vi "App - analyze RUS V6.vi"() -> ()   [LabVIEW 2021] (continued)
"last mod"=timestamp(3493899198 s since 1904-01-01), "file name str"="D:\\Data\\Ultrasound\\LSCO\\LSCO22__130814c\\5_Cooling_2nd_try\\September_2014\\091814\\14.78800K_500_2500_2.10000V_0.00000T_Sep18-2014__11-33-18_001_091814.bin", "mod time(min)"=58231653.3, "file format"=enum."binary", "power(V)"=2.1, "Magn Field(T) "=0.0}, {"temperature"=14.791, "temperature str"="14.79100", "file path"=path "D:/Data/Ultrasound/LSCO/LSCO22__130814c/5_Cooling_2nd_try/September_2014/091814/14.79100K_500_2500_2.10000V_0.00000T_Sep18-2014__11-34-37_001_091814.bin", "last mod"=timestamp(3493899277 s since 1904-01-01), "file name str"="D:\\Data\\Ultrasound\\LSCO\\LSCO22__130814c\\5_Cooling_2nd_try\\September_2014\\091814\\14.79100K_500_2500_2.10000V_0.00000T_Sep18-2014__11-34-37_001_091814.bin", "mod time(min)"=58231654.61666667, "file format"=enum."binary", "power(V)"=2.1, "Magn Field(T) "=0.0}, {"temperature"=14.793, "temperature str"="14.79300", "file path"=path "D:/Data/Ultrasound/LSCO/LSCO22__130814c/5_Cooling_2nd_try/September_2014/091814/14.79300K_500_2500_2.10000V_0.00000T_Sep18-2014__11-35-56_001_091814.bin", "last mod"=timestamp(3493899356 s since 1904-01-01), "file name str"="D:\\Data\\Ultrasound\\LSCO\\LSCO22__130814c\\5_Cooling_2nd_try\\September_2014\\091814\\14.79300K_500_2500_2.10000V_0.00000T_Sep18-2014__11-35-56_001_091814.bin", "mod time(min)"=58231655.93333333, "file format"=enum."binary", "power(V)"=2.1, "Magn Field(T) "=0.0}, {"temperature"=14.796, "temperature str"="14.79600", "file path"=path "D:/Data/Ultrasound/LSCO/LSCO22__130814c/5_Cooling_2nd_try/September_2014/091814/14.79600K_500_2500_2.10000V_0.00000T_Sep18-2014__11-37-16_001_091814.bin", "last mod"=timestamp(3493899436 s since 1904-01-01), "file name str"="D:\\Data\\Ultrasound\\LSCO\\LSCO22__130814c\\5_Cooling_2nd_try\\September_2014\\091814\\14.79600K_500_2500_2.10000V_0.00000T_Sep18-2014__11-37-16_001_091814.bin", "mod time(min)"=58231657.266666666, "file format"=enum."binary", "power(V)"=2.1, "Magn Field(T) "=0.0}, {"temperature"=14.797, "temperature str"="14.79700", "file path"=path "D:/Data/Ultrasound/LSCO/LSCO22__130814c/5_Cooling_2nd_try/September_2014/091814/14.79700K_500_2500_2.10000V_0.00000T_Sep18-2014__11-38-35_001_091814.bin", "last mod"=timestamp(3493899515 s since 1904-01-01), "file name str"="D:\\Data\\Ultrasound\\LSCO\\LSCO22__130814c\\5_Cooling_2nd_try\\September_2014\\091814\\14.79700K_500_2500_2.10000V_0.00000T_Sep18-2014__11-38-35_001_091814.bin", "mod time(min)"=58231658.583333336, "file format"=enum."binary", "power(V)"=2.1, "Magn Field(T) "=0.0}, {"temperature"=14.8, "temperature str"="14.80000", "file path"=path "D:/Data/Ultrasound/LSCO/LSCO22__130814c/5_Cooling_2nd_try/September_2014/091814/14.80000K_500_2500_2.10000V_0.00000T_Sep18-2014__11-39-54_001_091814.bin", "last mod"=timestamp(3493899594 s since 1904-01-01), "file name str"="D:\\Data\\Ultrasound\\LSCO\\LSCO22__130814c\\5_Cooling_2nd_try\\September_2014\\091814\\14.80000K_500_2500_2.10000V_0.00000T_Sep18-2014__11-39-54_001_091814.bin", "mod time(min)"=58231659.9, "file format"=enum."binary", "power(V)"=2.1, "Magn Field(T) "=0.0}, {"temperature"=14.807, "temperature str"="14.80700", "file path"=path "D:/Data/Ultrasound/LSCO/LSCO22__130814c/5_Cooling_2nd_try/September_2014/091814/14.80700K_500_2500_2.10000V_0.00000T_Sep18-2014__11-41-14_001_091814.bin", "last mod"=timestamp(3493899674 s since 1904-01-01), "file name str"="D:\\Data\\Ultrasound\\LSCO\\LSCO22__130814c\\5_Cooling_2nd_try\\September_2014\\091814\\14.80700K_500_2500_2.10000V_0.00000T_Sep18-2014__11-41-14_001_091814.bin", "mod time(min)"=58231661.233333334, "file format"=enum."binary", "power(V)"=2.1, "Magn Field(T) "=0.0}, {"temperature"=14.806, "temperature str"="14.80600", "file path"=path "D:/Data/Ultrasound/LSCO/LSCO22__130814c/5_Cooling_2nd_try/September_2014/091814/14.80600K_500_2500_2.10000V_0.00000T_Sep18-2014__11-42-33_001_091814.bin", "last mod"=timestamp(3493899753 s since 1904-01-01), "file name str"="D:\\Data\\Ultrasound\\LSCO\\LSCO22__130814c\\5_Cooling_2nd_try\\September_2014\\091814\\14.80600K_500_2500_2.10000V_0.00000T_Sep18-2014__11-42-33_001_091814.bin", "mod time(min)"=58231662.55, "file format"=enum."binary", "power(V)"=2.1, "Magn Field(T) "=0.0}, {"temperature"=14.808, "temperature str"="14.80800", "file path"=path "D:/Data/Ultrasound/LSCO/LSCO22__130814c/5_Cooling_2nd_try/September_2014/091814/14.80800K_500_2500_2.10000V_0.00000T_Sep18-2014__11-43-53_001_091814.bin", "last mod"=timestamp(3493899833 s since 1904-01-01), "file name str"="D:\\Data\\Ultrasound\\LSCO\\LSCO22__130814c\\5_Cooling_2nd_try\\September_2014\\091814\\14.80800K_500_2500_2.10000V_0.00000T_Sep18-2014__11-43-53_001_091814.bin", "mod time(min)"=58231663.88333333, "file format"=enum."binary", "power(V)"=2.1, "Magn Field(T) "=0.0}, {"temperature"=14.812, "temperature str"="14.81200", "file path"=path "D:/Data/Ultrasound/LSCO/LSCO22__130814c/5_Cooling_2nd_try/September_2014/091814/14.81200K_500_2500_2.10000V_0.00000T_Sep18-2014__11-45-12_001_091814.bin", "last mod"=timestamp(3493899912 s since 1904-01-01), "file name str"="D:\\Data\\Ultrasound\\LSCO\\LSCO22__130814c\\5_Cooling_2nd_try\\September_2014\\091814\\14.81200K_500_2500_2.10000V_0.00000T_Sep18-2014__11-45-12_001_091814.bin", "mod time(min)"=58231665.2, "file format"=enum."binary", "power(V)"=2.1, "Magn Field(T) "=0.0}, {"temperature"=14.814, "temperature str"="14.81400", "file path"=path "D:/Data/Ultrasound/LSCO/LSCO22__130814c/5_Cooling_2nd_try/September_2014/091814/14.81400K_500_2500_2.10000V_0.00000T_Sep18-2014__11-46-31_001_091814.bin", "last mod"=timestamp(3493899991 s since 1904-01-01), "file name str"="D:\\Data\\Ultrasound\\LSCO\\LSCO22__130814c\\5_Cooling_2nd_try\\September_2014\\091814\\14.81400K_500_2500_2.10000V_0.00000T_Sep18-2014__11-46-31_001_091814.bin", "mod time(min)"=58231666.516666666, "file format"=enum."binary", "power(V)"=2.1, "Magn Field(T) "=0.0}, {"temperature"=14.82, "temperature str"="14.82000", "file path"=path "D:/Data/Ultrasound/LSCO/LSCO22__130814c/5_Cooling_2nd_try/September_2014/091814/14.82000K_500_2500_2.10000V_0.00000T_Sep18-2014__11-47-51_001_091814.bin", "last mod"=timestamp(3493900071 s since 1904-01-01), "file name str"="D:\\Data\\Ultrasound\\LSCO\\LSCO22__130814c\\5_Cooling_2nd_try\\September_2014\\091814\\14.82000K_500_2500_2.10000V_0.00000T_Sep18-2014__11-47-51_001_091814.bin", "mod time(min)"=58231667.85, "file format"=enum."binary", "power(V)"=2.1, "Magn Field(T) "=0.0}, {"temperature"=14.816, "temperature str"="14.81600", "file path"=path "D:/Data/Ultrasound/LSCO/LSCO22__130814c/5_Cooling_2nd_try/September_2014/091814/14.81600K_500_2500_2.10000V_0.00000T_Sep18-2014__11-49-10_001_091814.bin", "last mod"=timestamp(3493900150 s since 1904-01-01), "file name str"="D:\\Data\\Ultrasound\\LSCO\\LSCO22__130814c\\5_Cooling_2nd_try\\September_2014\\091814\\14.81600K_500_2500_2.10000V_0.00000T_Sep18-2014__11-49-10_001_091814.bin", "mod time(min)"=58231669.166666664, "file format"=enum."binary", "power(V)"=2.1, "Magn Field(T) "=0.0}]
  out "freqout file":path=path "D:/Data/Ultrasound/LSCO/LSCO22__130814c/5_Cooling_2nd_try/9w/664_a.dat"
  out "lorentzian points":T27[](array[typedef])=[{"temperature"=241.719, "lorentzian"={"A (VHz)"=0.0, "ω (Hz)"=0.0, "Γ (Hz)"=0.0, "φ (rad)"=0.0, "Q"=0.0, "Norm  Ampl"=0.0, "z∞ (V)"=0.0+0.0i, "4corners"={"z (-pi/2)"=0.0+0.0i, "z(inf)"=0.0+0.0i, "z (pi/2)"=0.0+0.0i, "z center"=0.0+0.0i, "z(0)"=0.0+0.0i, "radius"=0.0}}, "timestamp(min)"=0.0, "timestamp"=timestamp(3493727821 s since 1904-01-01), "Magn Field(T)"=0.0}, {"temperature"=220.002, "lorentzian"={"A (VHz)"=0.0, "ω (Hz)"=0.0, "Γ (Hz)"=0.0, "φ (rad)"=0.0, "Q"=0.0, "Norm  Ampl"=0.0, "z∞ (V)"=0.0+0.0i, "4corners"={"z (-pi/2)"=0.0+0.0i, "z(inf)"=0.0+0.0i, "z (pi/2)"=0.0+0.0i, "z center"=0.0+0.0i, "z(0)"=0.0+0.0i, "radius"=0.0}}, "timestamp(min)"=21.30000000447035, "timestamp"=timestamp(3493729099 s since 1904-01-01), "Magn Field(T)"=0.0}, {"temperature"=219.999, "lorentzian"={"A (VHz)"=0.0, "ω (Hz)"=0.0, "Γ (Hz)"=0.0, "φ (rad)"=0.0, "Q"=0.0, "Norm  Ampl"=0.0, "z∞ (V)"=0.0+0.0i, "4corners"={"z (-pi/2)"=0.0+0.0i, "z(inf)"=0.0+0.0i, "z (pi/2)"=0.0+0.0i, "z center"=0.0+0.0i, "z(0)"=0.0+0.0i, "radius"=0.0}}, "timestamp(min)"=23.58333333581686, "timestamp"=timestamp(3493729236 s since 1904-01-01), "Magn Field(T)"=0.0}, {"temperature"=220.002, "lorentzian"={"A (VHz)"=0.0, "ω (Hz)"=0.0, "Γ (Hz)"=0.0, "φ (rad)"=0.0, "Q"=0.0, "Norm  Ampl"=0.0, "z∞ (V)"=0.0+0.0i, "4corners"={"z (-pi/2)"=0.0+0.0i, "z(inf)"=0.0+0.0i, "z (pi/2)"=0.0+0.0i, "z center"=0.0+0.0i, "z(0)"=0.0+0.0i, "radius"=0.0}}, "timestamp(min)"=24.91666666418314, "timestamp"=timestamp(3493729316 s since 1904-01-01), "Magn Field(T)"=0.0}, {"temperature"=221.376, "lorentzian"={"A (VHz)"=0.0, "ω (Hz)"=0.0, "Γ (Hz)"=0.0, "φ (rad)"=0.0, "Q"=0.0, "Norm  Ampl"=0.0, "z∞ (V)"=0.0+0.0i, "4corners"={"z (-pi/2)"=0.0+0.0i, "z(inf)"=0.0+0.0i, "z (pi/2)"=0.0+0.0i, "z center"=0.0+0.0i, "z(0)"=0.0+0.0i, "radius"=0.0}}, "timestamp(min)"=26.233333334326744, "timestamp"=timestamp(3493729395 s since 1904-01-01), "Magn Field(T)"=0.0}, {"temperature"=220.736, "lorentzian"={"A (VHz)"=0.0, "ω (Hz)"=0.0, "Γ (Hz)"=0.0, "φ (rad)"=0.0, "Q"=0.0, "Norm  Ampl"=0.0, "z∞ (V)"=0.0+0.0i, "4corners"={"z (-pi/2)"=0.0+0.0i, "z(inf)"=0.0+0.0i, "z (pi/2)"=0.0+0.0i, "z center"=0.0+0.0i, "z(0)"=0.0+0.0i, "radius"=0.0}}, "timestamp(min)"=27.566666670143604, "timestamp"=timestamp(3493729475 s since 1904-01-01), "Magn Field(T)"=0.0}, {"temperature"=220.112, "lorentzian"={"A (VHz)"=0.0, "ω (Hz)"=0.0, "Γ (Hz)"=0.0, "φ (rad)"=0.0, "Q"=0.0, "Norm  Ampl"=0.0, "z∞ (V)"=0.0+0.0i, "4corners"={"z (-pi/2)"=0.0+0.0i, "z(inf)"=0.0+0.0i, "z (pi/2)"=0.0+0.0i, "z center"=0.0+0.0i, "z(0)"=0.0+0.0i, "radius"=0.0}}, "timestamp(min)"=28.883333332836628, "timestamp"=timestamp(3493729554 s since 1904-01-01), "Magn Field(T)"=0.0}, {"temperature"=219.885, "lorentzian"={"A (VHz)"=0.0, "ω (Hz)"=0.0, "Γ (Hz)"=0.0, "φ (rad)"=0.0, "Q"=0.0, "Norm  Ampl"=0.0, "z∞ (V)"=0.0+0.0i, "4corners"={"z (-pi/2)"=0.0+0.0i, "z(inf)"=0.0+0.0i, "z (pi/2)"=0.0+0.0i, "z center"=0.0+0.0i, "z(0)"=0.0+0.0i, "radius"=0.0}}, "timestamp(min)"=30.200000002980232, "timestamp"=timestamp(3493729633 s since 1904-01-01), "Magn Field(T)"=0.0}, {"temperature"=219.907, "lorentzian"={"A (VHz)"=0.0, "ω (Hz)"=0.0, "Γ (Hz)"=0.0, "φ (rad)"=0.0, "Q"=0.0, "Norm  Ampl"=0.0, "z∞ (V)"=0.0+0.0i, "4corners"={"z (-pi/2)"=0.0+0.0i, "z(inf)"=0.0+0.0i, "z (pi/2)"=0.0+0.0i, "z center"=0.0+0.0i, "z(0)"=0.0+0.0i, "radius"=0.0}}, "timestamp(min)"=31.533333331346512, "timestamp"=timestamp(3493729713 s since 1904-01-01), "Magn Field(T)"=0.0}, {"temperature"=220.061, "lorentzian"={"A (VHz)"=0.0, "ω (Hz)"=0.0, "Γ (Hz)"=0.0, "φ (rad)"=0.0, "Q"=0.0, "Norm  Ampl"=0.0, "z∞ (V)"=0.0+0.0i, "4corners"={"z (-pi/2)"=0.0+0.0i, "z(inf)"=0.0+0.0i, "z (pi/2)"=0.0+0.0i, "z center"=0.0+0.0i, "z(0)"=0.0+0.0i, "radius"=0.0}}, "timestamp(min)"=32.850000001490116, "timestamp"=timestamp(3493729792 s since 1904-01-01), "Magn Field(T)"=0.0}, {"temperature"=220.167, "lorentzian"={"A (VHz)"=0.0, "ω (Hz)"=0.0, "Γ (Hz)"=0.0, "φ (rad)"=0.0, "Q"=0.0, "Norm  Ampl"=0.0, "z∞ (V)"=0.0+0.0i, "4corners"={"z (-pi/2)"=0.0+0.0i, "z(inf)"=0.0+0.0i, "z (pi/2)"=0.0+0.0i, "z center"=0.0+0.0i, "z(0)"=0.0+0.0i, "radius"=0.0}}, "timestamp(min)"=34.16666666418314, "timestamp"=timestamp(3493729871 s since 1904-01-01), "Magn Field(T)"=0.0}, {"temperature"=220.232, "lorentzian"={"A (VHz)"=0.0, "ω (Hz)"=0.0, "Γ (Hz)"=0.0, "φ (rad)"=0.0, "Q"=0.0, "Norm  Ampl"=0.0, "z∞ (V)"=0.0+0.0i, "4corners"={"z (-pi/2)"=0.0+0.0i, "z(inf)"=0.0+0.0i, "z (pi/2)"=0.0+0.0i, "z center"=0.0+0.0i, "z(0)"=0.0+0.0i, "radius"=0.0}}, "timestamp(min)"=35.5, "timestamp"=timestamp(3493729951 s since 1904-01-01), "Magn Field(T)"=0.0}, {"temperature"=220.32, "lorentzian"={"A (VHz)"=0.0, "ω (Hz)"=0.0, "Γ (Hz)"=0.0, "φ (rad)"=0.0, "Q"=0.0, "Norm  Ampl"=0.0, "z∞ (V)"=0.0+0.0i, "4corners"={"z (-pi/2)"=0.0+0.0i, "z(inf)"=0.0+0.0i, "z (pi/2)"=0.0+0.0i, "z center"=0.0+0.0i, "z(0)"=0.0+0.0i, "radius"=0.0}}, "timestamp(min)"=36.816666670143604, "timestamp"=timestamp(3493730030 s since 1904-01-01), "Magn Field(T)"=0.0}, {"temperature"=220.447, "lorentzian"={"A (VHz)"=0.0, "ω (Hz)"=0.0, "Γ (Hz)"=0.0, "φ (rad)"=0.0, "Q"=0.0, "Norm  Ampl"=0.0, "z∞ (V)"=0.0+0.0i, "4corners"={"z (-pi/2)"=0.0+0.0i, "z(inf)"=0.0+0.0i, "z (pi/2)"=0.0+0.0i, "z center"=0.0+0.0i, "z(0)"=0.0+0.0i, "radius"=0.0}}, "timestamp(min)"=38.149999998509884, "timestamp"=timestamp(3493730110 s since 1904-01-01), "Magn Field(T)"=0.0}, {"temperature"=220.033, "lorentzian"={"A (VHz)"=0.0, "ω (Hz)"=0.0, "Γ (Hz)"=0.0, "φ (rad)"=0.0, "Q"=0.0, "Norm  Ampl"=0.0, "z∞ (V)"=0.0+0.0i, "4corners"={"z (-pi/2)"=0.0+0.0i, "z(inf)"=0.0+0.0i, "z (pi/2)"=0.0+0.0i, "z center"=0.0+0.0i, "z(0)"=0.0+0.0i, "radius"=0.0}}, "timestamp(min)"=39.46666666865349, "timestamp"=timestamp(3493730189 s since 1904-01-01), "Magn Field(T)"=0.0}, {"temperature"=219.225, "lorentzian"={"A (VHz)"=0.0, "ω (Hz)"=0.0, "Γ (Hz)"=0.0, "φ (rad)"=0.0, "Q"=0.0, "Norm  Ampl"=0.0, "z∞ (V)"=0.0+0.0i, "4corners"={"z (-pi/2)"=0.0+0.0i, "z(inf)"=0.0+0.0i, "z (pi/2)"=0.0+0.0i, "z center"=0.0+0.0i, "z(0)"=0.0+0.0i, "radius"=0.0}}, "timestamp(min)"=40.78333333134651, "timestamp"=timestamp(3493730268 s since 1904-01-01), "Magn Field(T)"=0.0}, {"temperature"=219.76, "lorentzian"={"A (VHz)"=0.0, "ω (Hz)"=0.0, "Γ (Hz)"=0.0, "φ (rad)"=0.0, "Q"=0.0, "Norm  Ampl"=0.0, "z∞ (V)"=0.0+0.0i, "4corners"={"z (-pi/2)"=0.0+0.0i, "z(inf)"=0.0+0.0i, "z (pi/2)"=0.0+0.0i, "z center"=0.0+0.0i, "z(0)"=0.0+0.0i, "radius"=0.0}}, "timestamp(min)"=42.11666666716337, "timestamp"=timestamp(3493730348 s since 1904-01-01), "Magn Field(T)"=0.0}, {"temperature"=220.195, "lorentzian"={"A (VHz)"=0.0, "ω (Hz)"=0.0, "Γ (Hz)"=0.0, "φ (rad)"=0.0, "Q"=0.0, "Norm  Ampl"=0.0, "z∞ (V)"=0.0+0.0i, "4corners"={"z (-pi/2)"=0.0+0.0i, "z(inf)"=0.0+0.0i, "z (pi/2)"=0.0+0.0i, "z center"=0.0+0.0i, "z(0)"=0.0+0.0i, "radius"=0.0}}, "timestamp(min)"=43.433333337306976, "timestamp"=timestamp(3493730427 s since 1904-01-01), "Magn Field(T)"=0.0}, {"temperature"=219.549, "lorentzian"={"A (VHz)"=0.0, "ω (Hz)"=0.0, "Γ (Hz)"=0.0, "φ (rad)"=0.0, "Q"=0.0, "Norm  Ampl"=0.0, "z∞ (V)"=0.0+0.0i, "4corners"={"z (-pi/2)"=0.0+0.0i, "z(inf)"=0.0+0.0i, "z (pi/2)"=0.0+0.0i, "z center"=0.0+0.0i, "z(0)"=0.0+0.0i, "radius"=0.0}}, "timestamp(min)"=44.75, "timestamp"=timestamp(3493730506 s since 1904-01-01), "Magn Field(T)"=0.0}, {"temperature"=219.085, "lorentzian"={"A (VHz)"=0.0, "ω (Hz)"=0.0, "Γ (Hz)"=0.0, "φ (rad)"=0.0, "Q"=0.0, "Norm  Ampl"=0.0, "z∞ (V)"=0.0+0.0i, "4corners"={"z (-pi/2)"=0.0+0.0i, "z(inf)"=0.0+0.0i, "z (pi/2)"=0.0+0.0i, "z center"=0.0+0.0i, "z(0)"=0.0+0.0i, "radius"=0.0}}, "timestamp(min)"=46.08333333581686, "timestamp"=timestamp(3493730586 s since 1904-01-01), "Magn Field(T)"=0.0}, {"temperature"=219.006, "lorentzian"={"A (VHz)"=0.0, "ω (Hz)"=0.0, "Γ (Hz)"=0.0, "φ (rad)"=0.0, "Q"=0.0, "Norm  Ampl"=0.0, "z∞ (V)"=0.0+0.0i, "4corners"={"z (-pi/2)"=0.0+0.0i, "z(inf)"=0.0+0.0i, "z (pi/2)"=0.0+0.0i, "z center"=0.0+0.0i, "z(0)"=0.0+0.0i, "radius"=0.0}}, "timestamp(min)"=47.399999998509884, "timestamp"=timestamp(3493730665 s since 1904-01-01), "Magn Field(T)"=0.0}, {"temperature"=218.791, "lorentzian"={"A (VHz)"=0.0, "ω (Hz)"=0.0, "Γ (Hz)"=0.0, "φ (rad)"=0.0, "Q"=0.0, "Norm  Ampl"=0.0, "z∞ (V)"=0.0+0.0i, "4corners"={"z (-pi/2)"=0.0+0.0i, "z(inf)"=0.0+0.0i, "z (pi/2)"=0.0+0.0i, "z center"=0.0+0.0i, "z(0)"=0.0+0.0i, "radius"=0.0}}, "timestamp(min)"=48.733333334326744, "timestamp"=timestamp(3493730745 s since 1904-01-01), "Magn Field(T)"=0.0}, {"temperature"=218.445, "lorentzian"={"A (VHz)"=0.0, "ω (Hz)"=0.0, "Γ (Hz)"=0.0, "φ (rad)"=0.0, "Q"=0.0, "Norm  Ampl"=0.0, "z∞ (V)"=0.0+0.0i, "4corners"={"z (-pi/2)"=0.0+0.0i, "z(inf)"=0.0+0.0i, "z (pi/2)"=0.0+0.0i, "z center"=0.0+0.0i, "z(0)"=0.0+0.0i, "radius"=0.0}}, "timestamp(min)"=50.05000000447035, "timestamp"=timestamp(3493730824 s since 1904-01-01), "Magn Field(T)"=0.0}, {"temperature"=218.177, "lorentzian"={"A (VHz)"=0.0, "ω (Hz)"=0.0, "Γ (Hz)"=0.0, "φ (rad)"=0.0, "Q"=0.0, "Norm  Ampl"=0.0, "z∞ (V)"=0.0+0.0i, "4corners"={"z (-pi/2)"=0.0+0.0i, "z(inf)"=0.0+0.0i, "z (pi/2)"=0.0+0.0i, "z center"=0.0+0.0i, "z(0)"=0.0+0.0i, "radius"=0.0}}, "timestamp(min)"=51.36666666716337, "timestamp"=timestamp(3493730903 s since 1904-01-01), "Magn Field(T)"=0.0}, {"temperature"=217.946, "lorentzian"={"A (VHz)"=0.0, "ω (Hz)"=0.0, "Γ (Hz)"=0.0, "φ (rad)"=0.0, "Q"=0.0, "Norm  Ampl"=0.0, "z∞ (V)"=0.0+0.0i, "4corners"={"z (-pi/2)"=0.0+0.0i, "z(inf)"=0.0+0.0i, "z (pi/2)"=0.0+0.0i, "z center"=0.0+0.0i, "z(0)"=0.0+0.0i, "radius"=0.0}}, "timestamp(min)"=52.70000000298023, "timestamp"=timestamp(3493730983 s since 1904-01-01), "Magn Field(T)"=0.0}, {"temperature"=217.689, "lorentzian"={"A (VHz)"=0.0, "ω (Hz)"=0.0, "Γ (Hz)"=0.0, "φ (rad)"=0.0, "Q"=0.0, "Norm  Ampl"=0.0, "z∞ (V)"=0.0+0.0i, "4corners"={"z (-pi/2)"=0.0+0.0i, "z(inf)"=0.0+0.0i, "z (pi/2)"=0.0+0.0i, "z center"=0.0+0.0i, "z(0)"=0.0+0.0i, "radius"=0.0}}, "timestamp(min)"=54.016666665673256, "timestamp"=timestamp(3493731062 s since 1904-01-01), "Magn Field(T)"=0.0}, {"temperature"=217.41, "lorentzian"={"A (VHz)"=0.0, "ω (Hz)"=0.0, "Γ (Hz)"=0.0, "φ (rad)"=0.0, "Q"=0.0, "Norm  Ampl"=0.0, "z∞ (V)"=0.0+0.0i, "4corners"={"z (-pi/2)"=0.0+0.0i, "z(inf)"=0.0+0.0i, "z (pi/2)"=0.0+0.0i, "z center"=0.0+0.0i, "z(0)"=0.0+0.0i, "radius"=0.0}}, "timestamp(min)"=55.33333333581686, "timestamp"=timestamp(3493731141 s since 1904-01-01), "Magn Field(T)"=0.0}, {"temperature"=217.145, "lorentzian"={"A (VHz)"=0.0, "ω (Hz)"=0.0, "Γ (Hz)"=0.0, "φ (rad)"=0.0, "Q"=0.0, "Norm  Ampl"=0.0, "z∞ (V)"=0.0+0.0i, "4corners"={"z (-pi/2)"=0.0+0.0i, "z(inf)"=0.0+0.0i, "z (pi/2)"=0.0+0.0i, "z center"=0.0+0.0i, "z(0)"=0.0+0.0i, "radius"=0.0}}, "timestamp(min)"=56.66666666418314, "timestamp"=timestamp(3493731221 s since 1904-01-01), "Magn Field(T)"=0.0}, {"temperature"=216.895, "lorentzian"={"A (VHz)"=0.0, "ω (Hz)"=0.0, "Γ (Hz)"=0.0, "φ (rad)"=0.0, "Q"=0.0, "Norm  Ampl"=0.0, "z∞ (V)"=0.0+0.0i, "4corners"={"z (-pi/2)"=0.0+0.0i, "z(inf)"=0.0+0.0i, "z (pi/2)"=0.0+0.0i, "z center"=0.0+0.0i, "z(0)"=0.0+0.0i, "radius"=0.0}}, "timestamp(min)"=57.983333334326744, "timestamp"=timestamp(3493731300 s since 1904-01-01), "Magn Field(T)"=0.0}, {"temperature"=216.629, "lorentzian"={"A (VHz)"=0.0, "ω (Hz)"=0.0, "Γ (Hz)"=0.0, "φ (rad)"=0.0, "Q"=0.0, "Norm  Ampl"=0.0, "z∞ (V)"=0.0+0.0i, "4corners"={"z (-pi/2)"=0.0+0.0i, "z(inf)"=0.0+0.0i, "z (pi/2)"=0.0+0.0i, "z center"=0.0+0.0i, "z(0)"=0.0+0.0i, "radius"=0.0}}, "timestamp(min)"=59.316666670143604, "timestamp"=timestamp(3493731380 s since 1904-01-01), "Magn Field(T)"=0.0}, {"temperature"=216.359, "lorentzian"={"A (VHz)"=0.0, "ω (Hz)"=0.0, "Γ (Hz)"=0.0, "φ (rad)"=0.0, "Q"=0.0, "Norm  Ampl"=0.0, "z∞ (V)"=0.0+0.0i, "4corners"={"z (-pi/2)"=0.0+0.0i, "z(inf)"=0.0+0.0i, "z (pi/2)"=0.0+0.0i, "z center"=0.0+0.0i, "z(0)"=0.0+0.0i, "radius"=0.0}}, "timestamp(min)"=60.63333333283663, "timestamp"=timestamp(3493731459 s since 1904-01-01), "Magn Field(T)"=0.0}, {"temperature"=216.106, "lorentzian"={"A (VHz)"=0.0, "ω (Hz)"=0.0, "Γ (Hz)"=0.0, "φ (rad)"=0.0, "Q"=0.0, "Norm  Ampl"=0.0, "z∞ (V)"=0.0+0.0i, "4corners"={"z (-pi/2)"=0.0+0.0i, "z(inf)"=0.0+0.0i, "z (pi/2)"=0.0+0.0i, "z center"=0.0+0.0i, "z(0)"=0.0+0.0i, "radius"=0.0}}, "timestamp(min)"=61.95000000298023, "timestamp"=timestamp(3493731538 s since 1904-01-01), "Magn Field(T)"=0.0}, {"temperature"=215.839, "lorentzian"={"A (VHz)"=0.0, "ω (Hz)"=0.0, "Γ (Hz)"=0.0, "φ (rad)"=0.0, "Q"=0.0, "Norm  Ampl"=0.0, "z∞ (V)"=0.0+0.0i, "4corners"={"z (-pi/2)"=0.0+0.0i, "z(inf)"=0.0+0.0i, "z (pi/2)"=0.0+0.0i, "z center"=0.0+0.0i, "z(0)"=0.0+0.0i, "radius"=0.0}}, "timestamp(min)"=63.28333333134651, "timestamp"=timestamp(3493731618 s since 1904-01-01), "Magn Field(T)"=0.0}, {"temperature"=215.585, "lorentzian"={"A (VHz)"=0.0, "ω (Hz)"=0.0, "Γ (Hz)"=0.0, "φ (rad)"=0.0, "Q"=0.0, "Norm  Ampl"=0.0, "z∞ (V)"=0.0+0.0i, "4corners"={"z (-pi/2)"=0.0+0.0i, "z(inf)"=0.0+0.0i, "z (pi/2)"=0.0+0.0i, "z center"=0.0+0.0i, "z(0)"=0.0+0.0i, "radius"=0.0}}, "timestamp(min)"=64.60000000149012, "timestamp"=timestamp(3493731697 s since 1904-01-01), "Magn Field(T)"=0.0}, {"temperature"=215.319, "lorentzian"={"A (VHz)"=0.0, "ω (Hz)"=0.0, "Γ (Hz)"=0.0, "φ (rad)"=0.0, "Q"=0.0, "Norm  Ampl"=0.0, "z∞ (V)"=0.0+0.0i, "4corners"={"z (-pi/2)"=0.0+0.0i, "z(inf)"=0.0+0.0i, "z (pi/2)"=0.0+0.0i, "z center"=0.0+0.0i, "z(0)"=0.0+0.0i, "radius"=0.0}}, "timestamp(min)"=65.91666666418314, "timestamp"=timestamp(3493731776 s since 1904-01-01), "Magn Field(T)"=0.0}, {"temperature"=215.053, "lorentzian"={"A (VHz)"=0.0, "ω (Hz)"=0.0, "Γ (Hz)"=0.0, "φ (rad)"=0.0, "Q"=0.0, "Norm  Ampl"=0.0, "z∞ (V)"=0.0+0.0i, "4corners"={"z (-pi/2)"=0.0+0.0i, "z(inf)"=0.0+0.0i, "z (pi/2)"=0.0+0.0i, "z center"=0.0+0.0i, "z(0)"=0.0+0.0i, "radius"=0.0}}, "timestamp(min)"=67.25, "timestamp"=timestamp(3493731856 s since 1904-01-01), "Magn Field(T)"=0.0}, {"temperature"=214.797, "lorentzian"={"A (VHz)"=0.0, "ω (Hz)"=0.0, "Γ (Hz)"=0.0, "φ (rad)"=0.0, "Q"=0.0, "Norm  Ampl"=0.0, "z∞ (V)"=0.0+0.0i, "4corners"={"z (-pi/2)"=0.0+0.0i, "z(inf)"=0.0+0.0i, "z (pi/2)"=0.0+0.0i, "z center"=0.0+0.0i, "z(0)"=0.0+0.0i, "radius"=0.0}}, "timestamp(min)"=68.5666666701436, "timestamp"=timestamp(3493731935 s since 1904-01-01), "Magn Field(T)"=0.0}, {"temperature"=214.531, "lorentzian"={"A (VHz)"=0.0, "ω (Hz)"=0.0, "Γ (Hz)"=0.0, "φ (rad)"=0.0, "Q"=0.0, "Norm  Ampl"=0.0, "z∞ (V)"=0.0+0.0i, "4corners"={"z (-pi/2)"=0.0+0.0i, "z(inf)"=0.0+0.0i, "z (pi/2)"=0.0+0.0i, "z center"=0.0+0.0i, "z(0)"=0.0+0.0i, "radius"=0.0}}, "timestamp(min)"=69.89999999850988, "timestamp"=timestamp(3493732015 s since 1904-01-01), "Magn Field(T)"=0.0}, {"temperature"=214.276, "lorentzian"={"A (VHz)"=0.0, "ω (Hz)"=0.0, "Γ (Hz)"=0.0, "φ (rad)"=0.0, "Q"=0.0, "Norm  Ampl"=0.0, "z∞ (V)"=0.0+0.0i, "4corners"={"z (-pi/2)"=0.0+0.0i, "z(inf)"=0.0+0.0i, "z (pi/2)"=0.0+0.0i, "z center"=0.0+0.0i, "z(0)"=0.0+0.0i, "radius"=0.0}}, "timestamp(min)"=71.21666666865349, "timestamp"=timestamp(3493732094 s since 1904-01-01), "Magn Field(T)"=0.0}, {"temperature"=214.01, "lorentzian"={"A (VHz)"=0.0, "ω (Hz)"=0.0, "Γ (Hz)"=0.0, "φ (rad)"=0.0, "Q"=0.0, "Norm  Ampl"=0.0, "z∞ (V)"=0.0+0.0i, "4corners"={"z (-pi/2)"=0.0+0.0i, "z(inf)"=0.0+0.0i, "z (pi/2)"=0.0+0.0i, "z center"=0.0+0.0i, "z(0)"=0.0+0.0i, "radius"=0.0}}, "timestamp(min)"=72.53333333134651, "timestamp"=timestamp(3493732173 s since 1904-01-01), "Magn Field(T)"=0.0}, {"temperature"=213.745, "lorentzian"={"A (VHz)"=0.0, "ω (Hz)"=0.0, "Γ (Hz)"=0.0, "φ (rad)"=0.0, "Q"=0.0, "Norm  Ampl"=0.0, "z∞ (V)"=0.0+0.0i, "4corners"={"z (-pi/2)"=0.0+0.0i, "z(inf)"=0.0+0.0i, "z (pi/2)"=0.0+0.0i, "z center"=0.0+0.0i, "z(0)"=0.0+0.0i, "radius"=0.0}}, "timestamp(min)"=73.86666666716337, "timestamp"=timestamp(3493732253 s since 1904-01-01), "Magn Field(T)"=0.0}, {"temperature"=213.49, "lorentzian"={"A (VHz)"=0.0, "ω (Hz)"=0.0, "Γ (Hz)"=0.0, "φ (rad)"=0.0, "Q"=0.0, "Norm  Ampl"=0.0, "z∞ (V)"=0.0+0.0i, "4corners"={"z (-pi/2)"=0.0+0.0i, "z(inf)"=0.0+0.0i, "z (pi/2)"=0.0+0.0i, "z center"=0.0+0.0i, "z(0)"=0.0+0.0i, "radius"=0.0}}, "timestamp(min)"=75.18333333730698, "timestamp"=timestamp(3493732332 s since 1904-01-01), "Magn Field(T)"=0.0}, {"temperature"=213.225, "lorentzian"={"A (VHz)"=0.0, "ω (Hz)"=0.0, "Γ (Hz)"=0.0, "φ (rad)"=0.0, "Q"=0.0, "Norm  Ampl"=0.0, "z∞ (V)"=0.0+0.0i, "4corners"={"z (-pi/2)"=0.0+0.0i, "z(inf)"=0.0+0.0i, "z (pi/2)"=0.0+0.0i, "z center"=0.0+0.0i, "z(0)"=0.0+0.0i, "radius"=0.0}}, "timestamp(min)"=76.5, "timestamp"=timestamp(3493732411 s since 1904-01-01), "Magn Field(T)"=0.0}, {"temperature"=212.968, "lorentzian"={"A (VHz)"=0.0, "ω (Hz)"=0.0, "Γ (Hz)"=0.0, "φ (rad)"=0.0, "Q"=0.0, "Norm  Ampl"=0.0, "z∞ (V)"=0.0+0.0i, "4corners"={"z (-pi/2)"=0.0+0.0i, "z(inf)"=0.0+0.0i, "z (pi/2)"=0.0+0.0i, "z center"=0.0+0.0i, "z(0)"=0.0+0.0i, "radius"=0.0}}, "timestamp(min)"=77.83333333581686, "timestamp"=timestamp(3493732491 s since 1904-01-01), "Magn Field(T)"=0.0}, {"temperature"=212.699, "lorentzian"={"A (VHz)"=0.0, "ω (Hz)"=0.0, "Γ (Hz)"=0.0, "φ (rad)"=0.0, "Q"=0.0, "Norm  Ampl"=0.0, "z∞ (V)"=0.0+0.0i, "4corners"={"z (-pi/2)"=0.0+0.0i, "z(inf)"=0.0+0.0i, "z (pi/2)"=0.0+0.0i, "z center"=0.0+0.0i, "z(0)"=0.0+0.0i, "radius"=0.0}}, "timestamp(min)"=79.14999999850988, "timestamp"=timestamp(3493732570 s since 1904-01-01), "Magn Field(T)"=0.0}, {"temperature"=212.433, "lorentzian"={"A (VHz)"=0.0, "ω (Hz)"=0.0, "Γ (Hz)"=0.0, "φ (rad)"=0.0, "Q"=0.0, "Norm  Ampl"=0.0, "z∞ (V)"=0.0+0.0i, "4corners"={"z (-pi/2)"=0.0+0.0i, "z(inf)"=0.0+0.0i, "z (pi/2)"=0.0+0.0i, "z center"=0.0+0.0i, "z(0)"=0.0+0.0i, "radius"=0.0}}, "timestamp(min)"=80.48333333432674, "timestamp"=timestamp(3493732650 s since 1904-01-01), "Magn Field(T)"=0.0}, {"temperature"=212.177, "lorentzian"={"A (VHz)"=0.0, "ω (Hz)"=0.0, "Γ (Hz)"=0.0, "φ (rad)"=0.0, "Q"=0.0, "Norm  Ampl"=0.0, "z∞ (V)"=0.0+0.0i, "4corners"={"z (-pi/2)"=0.0+0.0i, "z(inf)"=0.0+0.0i, "z (pi/2)"=0.0+0.0i, "z center"=0.0+0.0i, "z(0)"=0.0+0.0i, "radius"=0.0}}, "timestamp(min)"=81.80000000447035, "timestamp"=timestamp(3493732729 s since 1904-01-01), "Magn Field(T)"=0.0}, {"temperature"=211.909, "lorentzian"={"A (VHz)"=0.0, "ω (Hz)"=0.0, "Γ (Hz)"=0.0, "φ (rad)"=0.0, "Q"=0.0, "Norm  Ampl"=0.0, "z∞ (V)"=0.0+0.0i, "4corners"={"z (-pi/2)"=0.0+0.0i, "z(inf)"=0.0+0.0i, "z (pi/2)"=0.0+0.0i, "z center"=0.0+0.0i, "z(0)"=0.0+0.0i, "radius"=0.0}}, "timestamp(min)"=83.11666666716337, "timestamp"=timestamp(3493732808 s since 1904-01-01), "Magn Field(T)"=0.0}, {"temperature"=211.653, "lorentzian"={"A (VHz)"=0.0003345488487757842, "ω (Hz)"=664.2436695290903, "Γ (Hz)"=0.17802124852951218, "φ (rad)"=-1.283320164921487, "Q"=3731.260593978885, "Norm  Ampl"=0.08412082785218908, "z∞ (V)"=0.48114096899499376+0.11397849685863293i, "4corners"={"z (-pi/2)"=0.16197849685863297-0.47314096899499375i, "z(inf)"=0.48114096899499376+0.11397849685863293i, "z (pi/2)"=-0.10597849685863292+0.4331409689949937i, "z center"=0.028000000000000025-0.020000000000000018i, "z(0)"=-0.4251409689949937-0.15397849685863296i, "radius"=0.47253251253455625}}, "timestamp(min)"=84.45000000298023, "timestamp"=timestamp(3493732888 s since 1904-01-01), "Magn Field(T)"=0.0}, {"temperature"=211.386, "lorentzian"={"A (VHz)"=0.0003397055053315072, "ω (Hz)"=664.2619309392137, "Γ (Hz)"=0.17590866140085512, "φ (rad)"=-1.2781485403251005, "Q"=3776.175235769173, "Norm  Ampl"=0.08254142638417036, "z∞ (V)"=0.4692788646297018+0.10736711353915548i, "4corners"={"z (-pi/2)"=0.15536711353915553-0.4772788646297018i, "z(inf)"=0.4692788646297018+0.10736711353915548i, "z (pi/2)"=-0.11536711353915549+0.42127886462970177i, "z center"=0.020000000000000018-0.028000000000000025i, "z(0)"=-0.4292788646297018-0.16336711353915553i, "radius"=0.4692288925789593}}, "timestamp(min)"=85.76666666567326, "timestamp"=timestamp(3493732967 s since 1904-01-01), "Magn Field(T)"=0.0}, {"temperature"=211.119, "lorentzian"={"A (VHz)"=0.00034204673996631043, "ω (Hz)"=664.2805728990513, "Γ (Hz)"=0.1744710249404492, "φ (rad)"=-1.2841598541798662, "Q"=3807.3976646023884, "Norm  Ampl"=0.08291010370324646, "z∞ (V)"=0.4758200604991372+0.1223545106284564i, "4corners"={"z (-pi/2)"=0.15435451062845643-0.4678200604991372i, 
